vi "DBLToString.vi"(0 "Number":dbl format="%#.20g", 5 "Precision":i16=6 caption="Precision (6)", 7 "Radix point":T1=enum."Comma (,)" caption="Radix point (,)", 9 "Remove trailing zeroes?":bool=TRUE caption="Remove trailing zeroes? (T)", 11 "Error in":errorcluster caption="Error in (no error)") -> (4 "String":string, 15 "Error out":errorcluster)   [LabVIEW 2017, in "GPString.lvlib"]
doc: "Converts <B>Number</B> to <B>String</B> observing the specified <B>Precision</B> and <B>Radix point</B>.\n\n<B>Radix point</B> can be either: System (localized), period (.), or comma (,).\n\nBy default this VI removes trailing zeroes in the fractional part. Set <B>Remove trailing zeroes?</B> to False if you want to keep <B>Precision</B> number of digits in the fractional part, even when the rightmost fractional digits are zeroes.\n\nThis VI is inlined and it runs only if there is no error on <B>Error in</B>.\n\nSteen Schmidt\nGPower\n25/9 2015"
uses:
  GPString.lvlib
  Typedefs/RadixPoint.ctl
panel:
  # "Copyright © 2015\nGPower\nSee enclosed license file for terms and conditions"
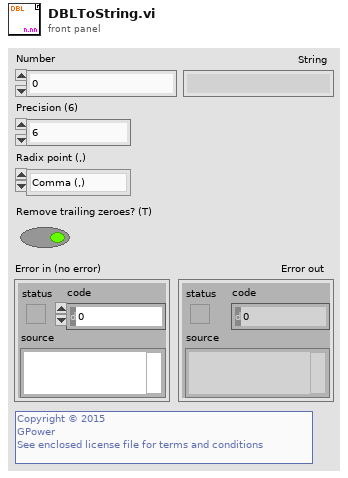
[diagram p1: front panel]
types:
  T1 = typedef "GPString.lvlib/RadixPoint.ctl" = enum16{"System", "Period (.)", "Comma (,)"}
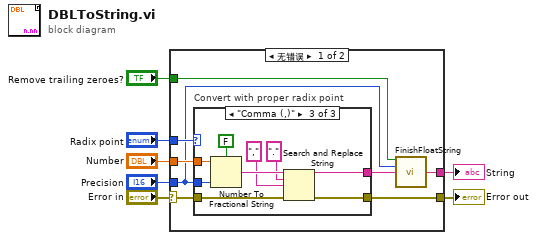
[diagram p0: block diagram]
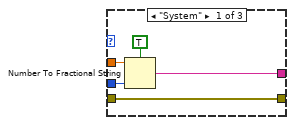
[diagram p2: hidden frame]
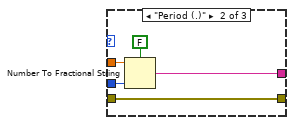
[diagram p3: hidden frame]
diagram:
  n1 = case shown="无错误" "Error in" {
    selector: "Error in" -> [w12 w35]
    tunnel: "Number" -> [w15 _]
    tunnel: "Precision" -> [w8 _]
    tunnel: "Radix point" -> [w14 _]
    tunnel: [w13 w35] -> w4
    tunnel: [w10 _] -> w3
    tunnel: "Remove trailing zeroes?" -> [w9 _]
    frame No Error {
      n2 = case "Convert with proper radix point" shown="\"Comma (,)\"" w14 {
        tunnel: w15 -> [w20 w25 w34]
        tunnel: w8 -> [w19 w24 w33]
        tunnel: [w18 w23 w30] -> w11
        tunnel: w12 -> [w16 w21 w27]
        tunnel: [w16 w21 w26] -> w13
        frame "System" {
          n3 = Number To Fractional String(use system decimal point (T)=TRUE, number=w20, precision (6)=w19) -> (F-format string=w18:string)  [unwired: 1 in]
        }
        frame "Period (.)" {
          n4 = Number To Fractional String(use system decimal point (T)=FALSE, number=w25, precision (6)=w24) -> (F-format string=w23:string)  [unwired: 1 in]
        }
        frame "Comma (,)" {
          n5 = Number To Fractional String(use system decimal point (T)=FALSE, number=w34, precision (6)=w33) -> (F-format string=w31:string)  [unwired: 1 in]
          n6 = Search and Replace String(input string=w31, search string=".", replace string="," ("search string"), error in=w27) -> (result string=w30:string, error out=w26:errorcluster)  [unwired: 4 in, 2 out]
        }
      }
      n7 = call "FinishFloatString.vi"("Remove trailing zeroes?"=w9, "Precision"=w8, "String"=w11) -> ("Finished string"=w10:string)  [unwired: 12 in]
    }
    frame Error {
    }
  }
  "String" <- w3
  "Error out" <- w4
